vi "Start.vi"(8 "error in (no error)":errorcluster, 11 "Framework in":refnum<class "Framework.lvclass">) -> (0 "error out":errorcluster, 3 "Framework out":refnum<class "Framework.lvclass">)   [LabVIEW 2017, in "DSF Core.lvlib" / "Framework.lvclass"]
uses:
  Framework.lvclass
  Framework.lvclass/Framework.ctl
  Thread Manager/Thread Manager.lvclass
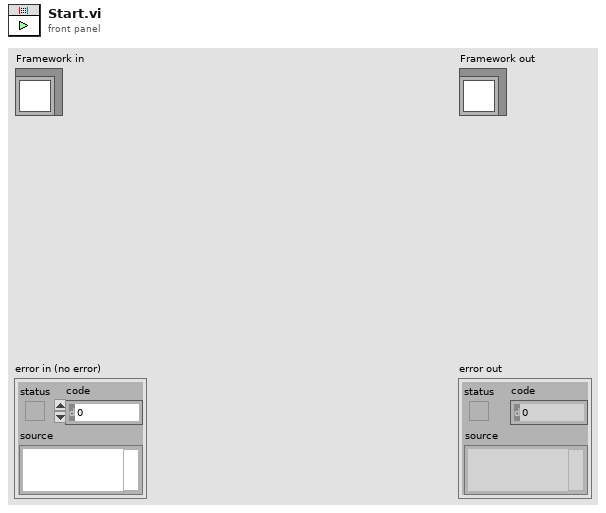
[diagram p1: front panel]
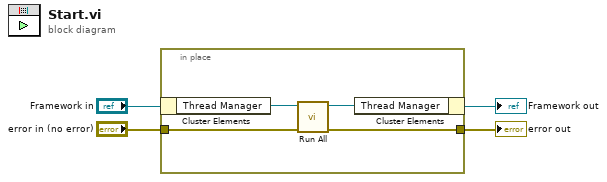
[diagram p0: block diagram]
diagram:
  n1 = in-place {
    in-place-border: "error in (no error)" -> [w8]
    in-place-border: [w6] -> w2
    n2 = in-place-cluster #1("Framework in") -> ("Thread Manager"=w7:refnum<class "Thread Manager.lvclass">)
    n3 = call "Run All.vi"("error in (no error)"=w8, "Thread Manager in"=w7) -> ("error out"=w6:errorcluster, "Thread Manager out"=w5:refnum<class "Thread Manager.lvclass">)  [unwired: 8 in]
    n4 = in-place-cluster #1("Thread Manager"=w5) -> (→"Framework out":refnum<class "Framework.lvclass">)
  }
  "error out" <- w2
